vi "Lab3_misure.vi"() -> ()   [LabVIEW 2024]
uses:
  <vilib>/Utility/error.llb/Trim Whitespace One-Sided.vi
  <vilib>/Instr/_visa.llb/VISA Configure Serial Port (Instr).vi
  <vilib>/Utility/file.llb/Write Delimited Spreadsheet (DBL).vi
panel:
  out "write buffer":string
  out "output 1":dbl
  out "read buffer":string
  out "Waveform Chart 2":dbl[](graph)
  in  "VISA resource name":refnum<visa-resource-name>
  out "Waveform Chart":T1(graph)
  out "?":dbl(slide) scale=0.0..40.0
  out "High":bool
  out "Ok":bool
  out "Low":bool
  out "Temperature  (°C)":dbl
  out "Conditioning (s)":dbl
  out "Heating (s)":dbl
  in  "Tmin (°C)":dbl
  in  "Tmax (°C)":dbl
  in  "?":bool
  in  "Knob simulating thermometer":dbl(knob) step=0.1 scale=10.0..40.0
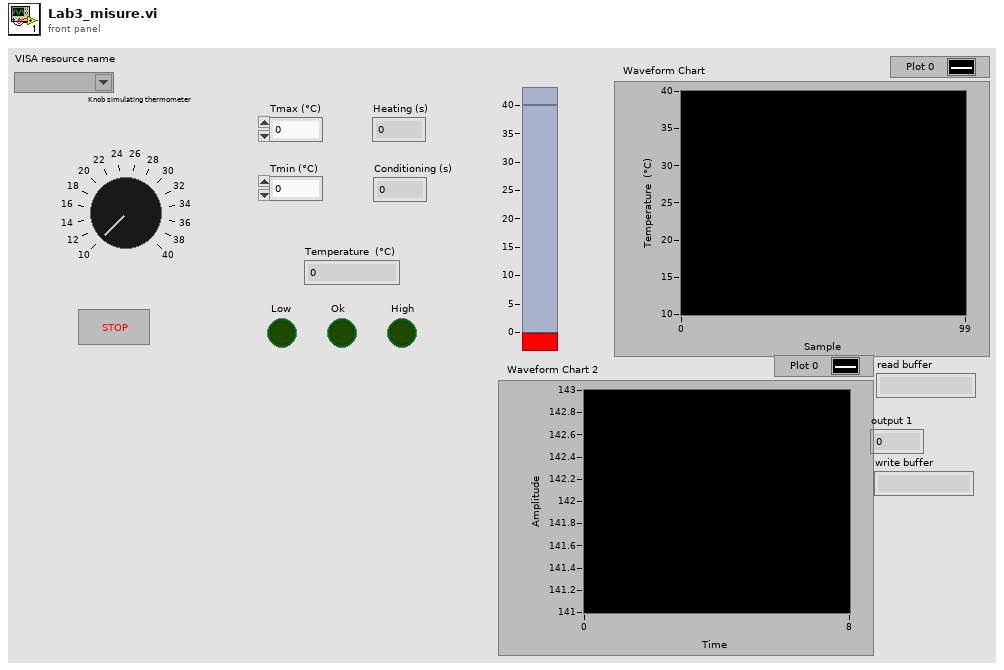
[diagram p1: front panel]
types:
  T1 = cluster{"Tmax (°C)":dbl, "Tmin (°C)":dbl, "Knob simulating thermometer":dbl}
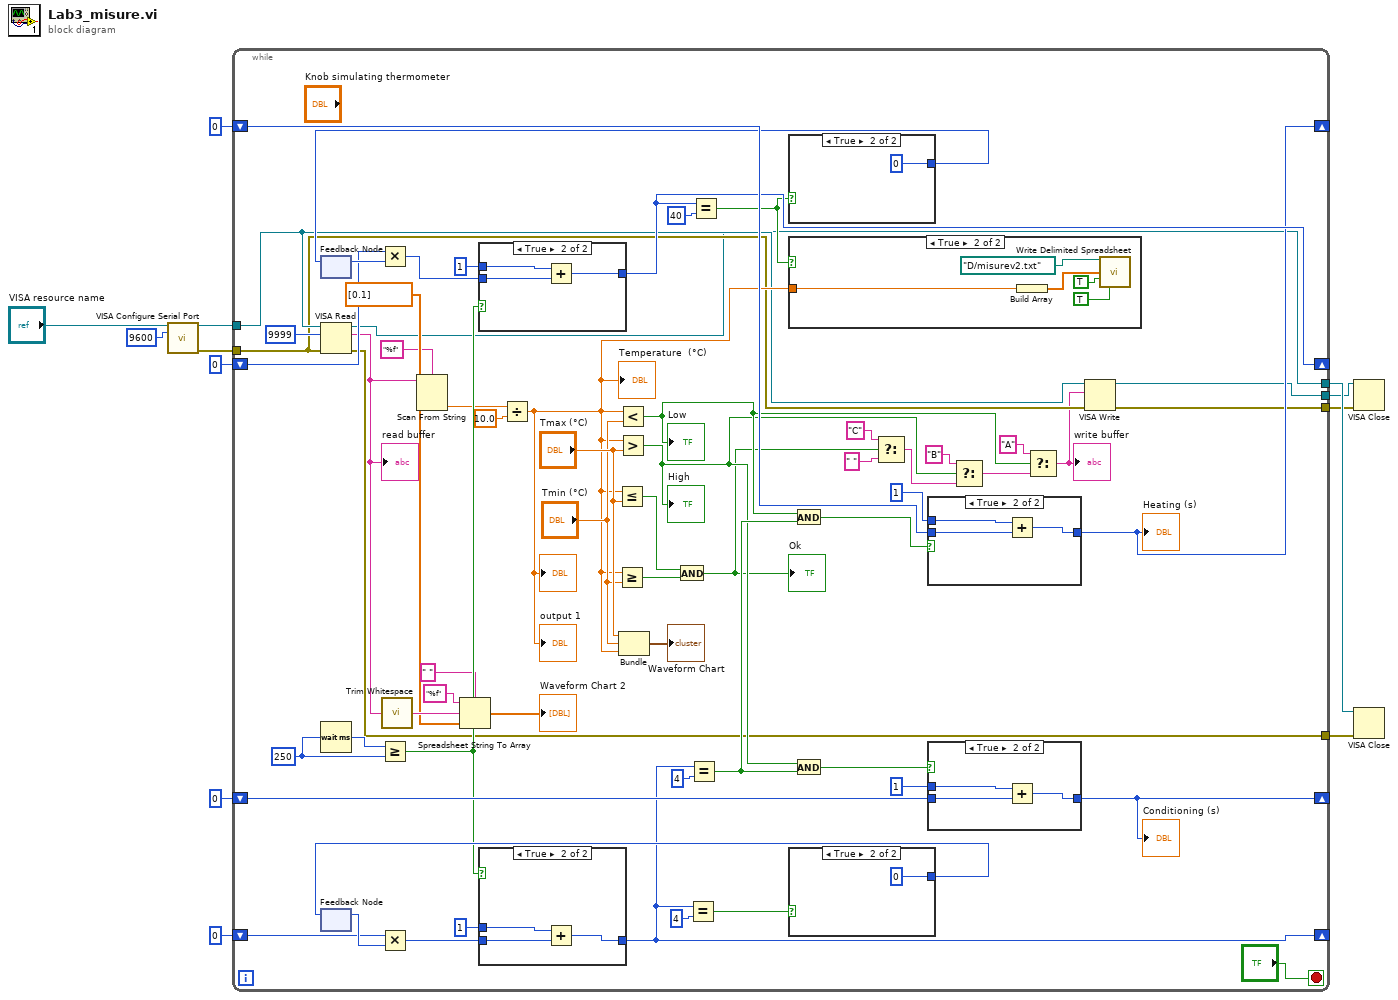
[diagram p0: block diagram]
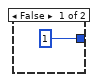
[diagram p2: hidden frame]
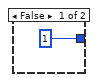
[diagram p4: hidden frame]
diagram:
  n1 = call-poly "VISA Configure Serial Port"("VISA resource name"="VISA resource name", "baud rate (9600)"=u32 9600) -> ("VISA resource name out"=w6:refnum<visa-resource-name>, "error out"=w5:errorcluster)  [unwired: 12 in]
  n2 = while {
    shift-right: [w58] -> _
    shift-left: 0 -> [w57]
    shift-right: [w42] -> _
    shift-left: 0 -> [w71]
    shift-right: [w54] -> _
    shift-left: 0 -> [w59]
    shift-right: [w44] -> _
    shift-left: 0 -> [w45]
    tunnel: w6 -> [w28]
    tunnel: w5 -> [w27]
    tunnel: [w16] -> w4
    tunnel: [w15] -> w3
    tunnel: [w14] -> w2
    tunnel: [w13] -> w1
    stop <- "?" stop-if-true
    w64 = 250
    n3 = feedback #1() -> (w48:i32)  [unwired: 1 in]
    n4 = VISA Read(VISA resource name=w28, byte count=u32 9999, error in (no error)=w27) -> (VISA resource name out=w15:refnum<visa-resource-name>, read buffer=w32:string, error out=w16:errorcluster)  [unwired: 1 out]
    "read buffer" <- w32
    n5 = Wait (ms)(milliseconds to wait=w64) -> (millisecond timer value=w65:u32)
    n6 = feedback #2() -> (w60:i32)  [unwired: 1 in]
    n7 = Multiply(x=w45, y=w48) -> (x*y=w50:i32)
    n8 = Greater Or Equal?(x=w65, y=w64) -> (x >= y?=w46:bool)
    n9 = Multiply(x=w59, y=w60) -> (x*y=w62:i32)
    n10 = call <vilib>:"Trim Whitespace.vi"("string"=w32) -> ("trimmed string"=w38:string)  [unwired: 1 in]
    n11 = Scan From String(format string="%f", input string=w32) -> (output 1=w31:dbl)  [unwired: 3 in, 3 out]
    n12 = Spreadsheet String To Array(delimiter (Tab)=" ", format string="%f", spreadsheet string=w38, array type (2D Dbl)=dbl[] [0.1]) -> (array=→"Waveform Chart 2":dbl[])
    n13 = case shown="True" w46 {
      tunnel: w50 -> [w77 w80]
      tunnel: [w77 w79] -> w44
      tunnel: 1 -> [_ w78]
      frame False {
      }
      frame True {
        n14 = Add(x=w78, y=w80) -> (x+y=w79:i32)
      }
    }
    n15 = case shown="True" w46 {
      tunnel: w62 -> [w83 w86]
      tunnel: [w83 w85] -> w54
      tunnel: 1 -> [_ w84]
      frame False {
      }
      frame True {
        n16 = Add(x=w84, y=w86) -> (x+y=w85:i32)
      }
    }
    n17 = Divide(x=w31, y=10.0) -> (x/y=w29:dbl)
    "Temperature  (°C)" <- w29
    "?" <- w29
    "output 1" <- w29
    n18 = Less Or Equal?(x=w29, y="Tmax (°C)") -> (x <= y?=w70:bool)
    n19 = Greater Or Equal?(x=w29, y="Tmin (°C)") -> (x >= y?=w69:bool)
    n20 = Less?(x=w29, y="Tmin (°C)") -> (x < y?=w26:bool)
    "Low" <- w26
    n21 = Greater?(x=w29, y="Tmax (°C)") -> (0:w24:bool)
    "High" <- w24
    n22 = Bundle("Tmax (°C)"="Tmax (°C)", "Tmin (°C)"="Tmin (°C)", w29) -> (→"Waveform Chart":cluster{"Tmax (°C)":dbl, "Tmin (°C)":dbl, dbl})  [unwired: 1 in]
    n23 = And(x=w70, y=w69) -> (x .and. y?=w22:bool)
    "Ok" <- w22
    n24 = Equal?(x=w54, y=4) -> (x = y?=w52:bool)
    n25 = Equal?(x=w54, y=4) -> (x = y?=w40:bool)
    n26 = Equal?(x=w44, y=40) -> (x = y?=w43:bool)
    n27 = case shown="True" w43 {
      tunnel: [1 0] -> w49
      frame False {
      }
      frame True {
      }
    }
    n28 = feedback-in #1(w49) -> ()
    n29 = case shown="True" w43 {
      tunnel: w29 -> [_ w87]
      frame False {
      }
      frame True {
        n30 = Build Array(w87) -> (w91:dbl[])
        n31 = call-poly <vilib>:"Write Delimited Spreadsheet.vi"("file path (dialog if empty)"=path "D:/misurev2.txt", "1D data"=w91, "append to file? (new file:F)"=TRUE, "transpose? (no:F)"=TRUE) -> ()  [unwired: 10 in, 2 out]
      }
    }
    n32 = case shown="True" w52 {
      tunnel: [1 0] -> w61
      frame False {
      }
      frame True {
      }
    }
    n33 = feedback-in #2(w61) -> ()
    n34 = And(x=w26, y=w40) -> (x .and. y?=w41:bool)
    n35 = And(x=w24, y=w40) -> (x .and. y?=w56:bool)
    n36 = Select(t="C" ("write buffer"), s=w22, f=" " ("write buffer")) -> (s? t:f=w19:string)
    n37 = case shown="True" w41 {
      tunnel: 1 -> [_ w95]
      tunnel: w71 -> [w92 w94]
      tunnel: [w92 w93] -> w42
      frame False {
      }
      frame True {
        n38 = Add(x=w95, y=w94) -> (x+y=w93:i32)
      }
    }
    "Heating (s)" <- w42
    n39 = case shown="True" w56 {
      tunnel: 1 -> [_ w99]
      tunnel: w57 -> [w96 w98]
      tunnel: [w96 w97] -> w58
      frame False {
      }
      frame True {
        n40 = Add(x=w99, y=w98) -> (x+y=w97:i32)
      }
    }
    "Conditioning (s)" <- w58
    n41 = Select(t="B" ("write buffer"), s=w24, f=w19) -> (s? t:f=w18:string)
    n42 = Select(t="A" ("write buffer"), s=w26, f=w18) -> (s? t:f=w17:string)
    "write buffer" <- w17
    n43 = VISA Write(VISA resource name=w28, write buffer=w17, error in (no error)=w27) -> (VISA resource name out=w13:refnum<visa-resource-name>, error out=w14:errorcluster)  [unwired: 1 out]
  }
  n44 = VISA Close(VISA resource name=w1, error in (no error)=w2) -> ()  [unwired: 1 out]
  n45 = VISA Close(VISA resource name=w3, error in (no error)=w4) -> ()  [unwired: 1 out]
